vi "TRAJECTORY_EXECUTE_REVERSE.vi"(5 "Wheel Base FT":dbl, 7 "Max Speed\nFT/SEC":dbl, 8 "Init":bool, 9 "Gyro Continous\n (inc counterclockwise)":dbl, 10 "Right Distance":dbl, 11 "Left Distance":dbl) -> (0 "AtReference":bool, 1 "Right Speed Target":dbl, 2 "Left Speed Target":dbl, 3 "outRAMSETE":T5={"B"=2.0, "Zeta"=0.7, "poseTolerance"={"TRANSLATION"={"X"=0.0, "Y"=0.0}, "ROTATION"={"VALUE"=0.0, "COS"=1.0, "SIN"=0.0}}, "poseError"={"TRANSLATION"={"X"=0.0, "Y"=0.0}, "ROTATION"={"VALUE"=0.0, "COS"=1.0, "SIN"=0.0}}, "Enabled"=TRUE} {"Zeta" format="%12.3f"; "B" format="%12.3f"}, 4 "CurrentRelativePose":T2, 6 "OutputTRAJ_STATE":T1={"TimeSeconds"=0.0, "Velocity"=0.0, "Acceleration"=0.0, "POSE"={"TRANSLATION"={"X"=0.0, "Y"=0.0}, "ROTATION"={"VALUE"=0.0, "COS"=1.0, "SIN"=0.0}}, "Curvature"=0.0})   [LabVIEW 2019]
uses:
  <vilib>/Rock Robotics/WPI/ThirdParty/JAS_Junk/TrajLib/POSE2D.ctl
  <vilib>/Rock Robotics/WPI/ThirdParty/JAS_Junk/TrajLib/TRANSLATION2D.ctl
  <vilib>/Rock Robotics/WPI/ThirdParty/JAS_Junk/TrajLib/ROTATION2D.ctl
  <vilib>/Rock Robotics/WPI/ThirdParty/JAS_Junk/TrajLib/RAMSETE.ctl
  <vilib>/Rock Robotics/WPI/ThirdParty/JAS_Junk/TrajLib/TRAJ_STATE.ctl
  <vilib>/Rock Robotics/WPI/ThirdParty/JAS_Junk/TrajLib/Rotation_CreateAngle.vi
  <vilib>/Rock Robotics/WPI/ThirdParty/JAS_Junk/TrajLib/Translation_Create.vi
  <vilib>/Rock Robotics/WPI/ThirdParty/JAS_Junk/TrajLib/Conv_Radians_Deg.vi
  <vilib>/Rock Robotics/WPI/ThirdParty/JAS_Junk/TrajLib/Trajectory_Library.lvlib
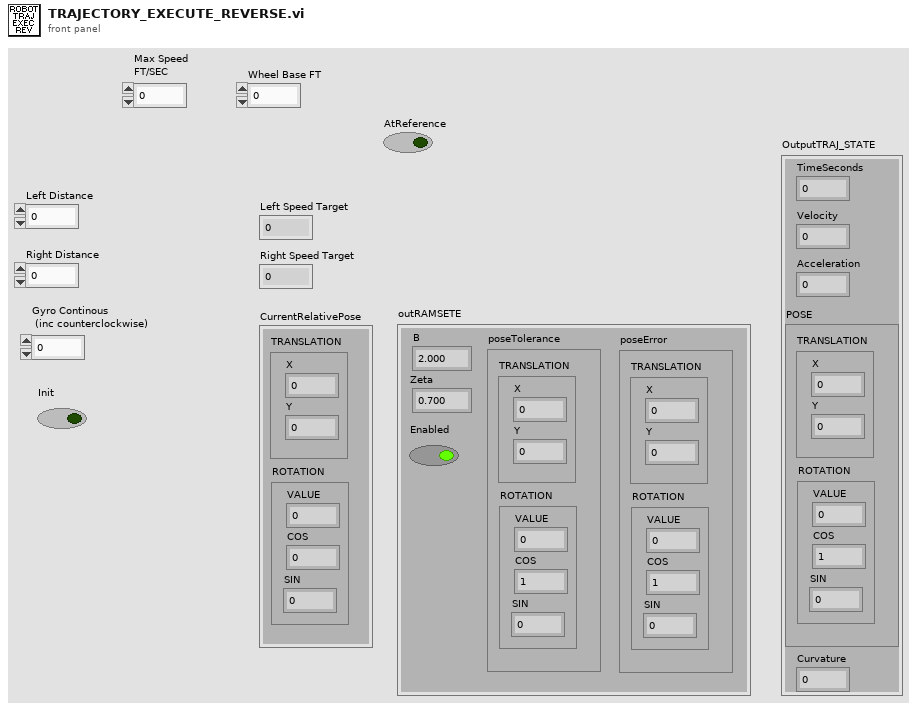
[diagram p1: front panel]
types:
  T1 = typedef "Trajectory_Library.lvlib/TRAJ_STATE.ctl" = cluster{"TimeSeconds":dbl, "Velocity":dbl, "Acceleration":dbl, "POSE":T2, "Curvature":dbl}
  T2 = typedef "Trajectory_Library.lvlib/POSE2D.ctl" = cluster{"TRANSLATION":T3, "ROTATION":T4}
  T3 = typedef "Trajectory_Library.lvlib/TRANSLATION2D.ctl" = cluster{"X":dbl, "Y":dbl}
  T4 = typedef "Trajectory_Library.lvlib/ROTATION2D.ctl" = cluster{"VALUE":dbl, "COS":dbl, "SIN":dbl}
  T5 = typedef "Trajectory_Library.lvlib/RAMSETE.ctl" = cluster{"B":dbl, "Zeta":dbl, "poseTolerance":T2, "poseError":T2, "Enabled":bool}
  T6 = typedef "Trajectory_Library.lvlib/TRAJECTORY.ctl" = cluster{"TotalTImeSecs":dbl, "States":T1[]}
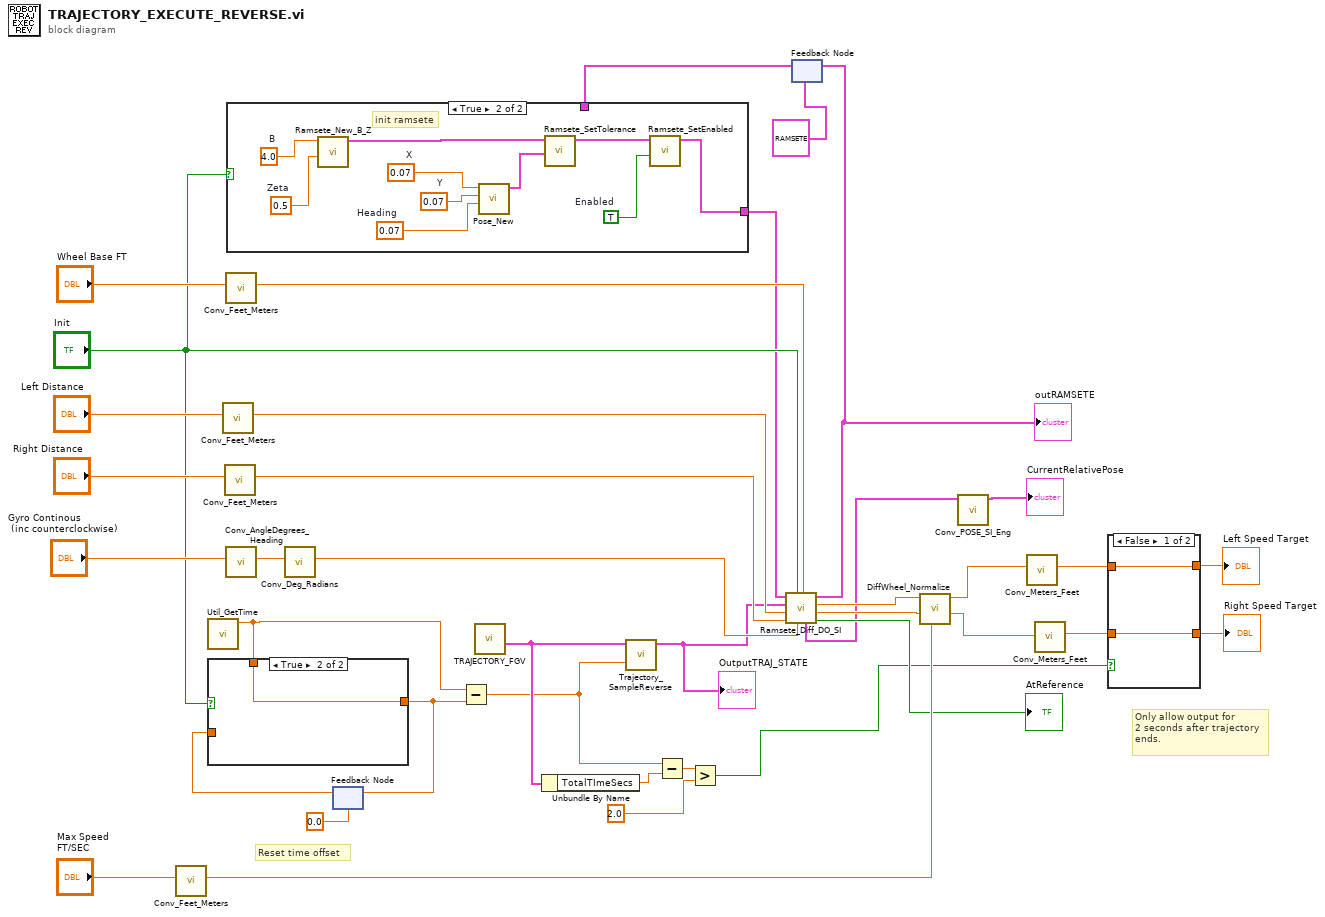
[diagram p0: block diagram]
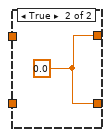
[diagram p3: hidden frame]
diagram:
  # "Only allow output for\n2 seconds after trajectory\nends."
  # "Reset time offset"
  n1 = call <vilib>:"Conv_Feet_Meters.vi"("Feet"="Max Speed\nFT/SEC") -> ("Meters"=w28:dbl)  [unwired: 10 in]
  n2 = call <vilib>:"Util_GetTime.vi"() -> ("FPGA_Time_Seconds"=w1:dbl)  [unwired: 11 in]
  n3 = call <vilib>:"Conv_Feet_Meters.vi"("Feet"="Left Distance") -> ("Meters"=w13:dbl)  [unwired: 10 in]
  n4 = call <vilib>:"Conv_Feet_Meters.vi"("Feet"="Right Distance") -> ("Meters"=w12:dbl)  [unwired: 10 in]
  n5 = call <vilib>:"Conv_Feet_Meters.vi"("Feet"="Wheel Base FT") -> ("Meters"=w10:dbl)  [unwired: 10 in]
  n6 = call <vilib>:"Conv_AngleDegrees_Heading.vi"("Degrees"="Gyro Continous\n (inc counterclockwise)") -> ("Heading Degrees"=w24:dbl)  [unwired: 10 in]
  n7 = call <vilib>:"Conv_Deg_Radians.vi"("Degress"=w24) -> ("Radians"=w11:dbl)  [unwired: 10 in]
  n8 = feedback #1(0.0 ("TIME")) -> (w37:dbl)
  n9 = case shown="True" "Init" {
    tunnel: [w39 w40] -> w36
    tunnel: w37 -> [w39 _]
    tunnel: w1 -> [_ w40]
    frame False {
    }
    frame True {
    }
  }
  n10 = feedback-in #1(w36) -> ()
  n11 = Subtract(x=w1, y=w36) -> (x-y=w21:dbl)
  n12 = call "TRAJECTORY_FGV.vi"() -> ("outTRAJECTORY"=w23:T6)  [unwired: 11 in]
  n13 = Unbundle By Name(w23) -> ("TotalTImeSecs"=w22:dbl)
  n14 = call <vilib>:"Trajectory_SampleReverse.vi"("Time"=w21, "InputTRAJECTORY"=w23) -> ("OutputTRAJ_STATE"=w2:T1)  [unwired: 9 in]
  "OutputTRAJ_STATE" <- w2
  n15 = Subtract(x=w21, y=w22) -> (x-y=w20:dbl)
  n16 = Greater?(x=w20, y=2.0) -> (0:w18:bool)
  n17 = feedback #2(T5 {"B"=2.0, "Zeta"=0.7, "poseTolerance"={"TRANSLATION"={"X"=0.0, "Y"=0.0}, "ROTATION"={"VALUE"=0.0, "COS"=1.0, "SIN"=0.0}}, "poseError"={"TRANSLATION"={"X"=0.0, "Y"=0.0}, "ROTATION"={"VALUE"=0.0, "COS"=1.0, "SIN"=0.0}}, "Enabled"=TRUE} ("RAMSETE")) -> (w7:T5)
  n18 = case shown="True" "Init" {
    tunnel: w7 -> [w41 _]
    tunnel: [w41 w49] -> w6
    frame False {
    }
    frame True {
      w42 = 0.5  # Zeta
      w43 = 4.0  # B
      w44 = 0.07  # Heading
      w45 = 0.07  # Y
      w46 = 0.07  # X
      w48 = TRUE  # Enabled
      # "init ramsete"
      n19 = call <vilib>:"Ramsete_New_B_Z.vi"("Zeta"=w42, "B"=w43) -> ("outRAMSETE"=w51:T5)  [unwired: 9 in]
      n20 = call <vilib>:"Pose_New.vi"("Heading"=w44, "Y"=w45, "X"=w46) -> ("out POSe"=w47:T2)  [unwired: 8 in]
      n21 = call <vilib>:"Ramsete_SetTolerance.vi"("tolerancePose"=w47, "inRAMSETE"=w51) -> ("outRAMSETE"=w50:T5)  [unwired: 9 in]
      n22 = call <vilib>:"Ramsete_SetEnabled.vi"("Enabled"=w48, "inRAMSETE"=w50) -> ("outRAMSETE"=w49:T5)  [unwired: 9 in]
    }
  }
  n23 = call <vilib>:"Ramsete_Diff_DO_SI.vi"("WheelBase-Meters"=w10, "Gyro-Radians"=w11, "Reset"="Init", "RightDist-Meters"=w12, "LeftDist-Meters"=w13, "TRAJ_STATE"=w2, "inRAMSETE"=w6) -> ("AtReference"=→"AtReference":bool, "RightVelDmd"=w29:dbl, "LeftVelDmd"=w30:dbl, "outRAMSETE"=w8:T5, "CurrentRelativePose"=w3:T2)
  "outRAMSETE" <- w8
  n24 = feedback-in #2(w8) -> ()
  n25 = call <vilib>:"DiffWheel_Normalize.vi"("Max Speed"=w28, "Right Wheel Demand"=w29, "Left Wheel Demand"=w30) -> ("Normalized Right Wheel Demand"=w25:dbl, "Normalized Left Wheel Demand"=w26:dbl)  [unwired: 7 in]
  n26 = call <vilib>:"Conv_POSE_SI_Eng.vi"("Err Pose in SI"=w3) -> ("Err Pose out ENG"=→"CurrentRelativePose":T2)  [unwired: 10 in]
  n27 = call <vilib>:"Conv_Meters_Feet.vi"("Meters"=w26) -> ("Feet"=w15:dbl)  [unwired: 10 in]
  n28 = call <vilib>:"Conv_Meters_Feet.vi"("Meters"=w25) -> ("Feet"=w14:dbl)  [unwired: 10 in]
  n29 = case shown="False" w18 {
    tunnel: [w53 w54] -> w17
    tunnel: [w52 w54] -> w16
    tunnel: w15 -> [w53 _]
    tunnel: w14 -> [w52 _]
    frame False {
    }
    frame True {
      w54 = 0.0
    }
  }
  "Left Speed Target" <- w17
  "Right Speed Target" <- w16
